vi "StateMachine.vi"() -> ()   [LabVIEW 2018]
panel:
  in  "정지":bool
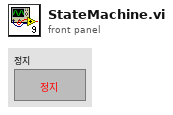
[diagram p1: front panel]
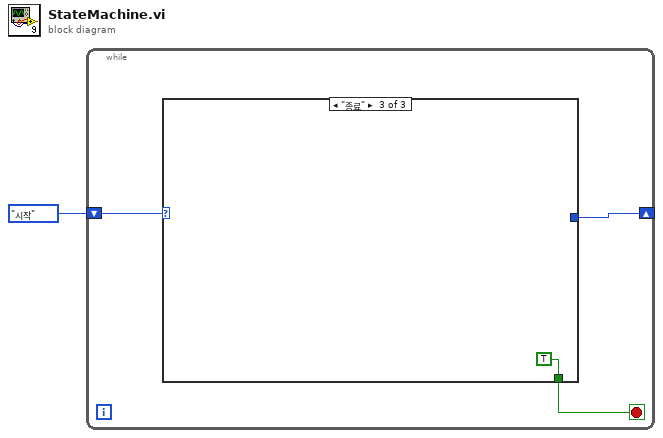
[diagram p0: block diagram]
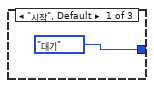
[diagram p2: hidden frame]
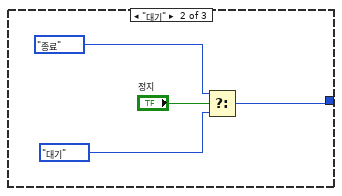
[diagram p3: hidden frame]
diagram:
  n1 = while {
    shift-right: [w3] -> _
    shift-left: enum16{"시작", "대기", "종료"}."시작" -> [w4]
    stop <- w2 stop-if-true
    n2 = case shown="\"종료\"" w4 {
      tunnel: [enum16{"시작", "대기", "종료"}."대기" w6 _] -> w3
      tunnel: [_ _ TRUE] -> w2
      frame "시작", Default {
      }
      frame "대기" {
        n3 = Select(t=enum16{"시작", "대기", "종료"}."종료", s="정지", f=enum16{"시작", "대기", "종료"}."대기") -> (s? t:f=w6:enum16{"시작", "대기", "종료"})
      }
      frame "종료" {
      }
    }
  }
